vi "CRYSelect result by name.vi"(10 "Result name desired":string, 11 "Result array":T2 {"Margin" format="%.2f"}) -> (0 "Exists?":bool, 3 "Desired Result":T1={"Name"="Test for Signal [L]", "Margin"=nan, "unit"="", "Verdict"=FALSE, "Limit"="", "Max/Min"="", "protected"=FALSE, "Step No."=0, "Test Info"="", "AutoProtect"=FALSE} {"Margin" format="%.2f"})   [LabVIEW 2013]
uses:
  Typedef Control/CRYResult Cluster Array.ctl
  Typedef Control/CRYResult Cluster.ctl
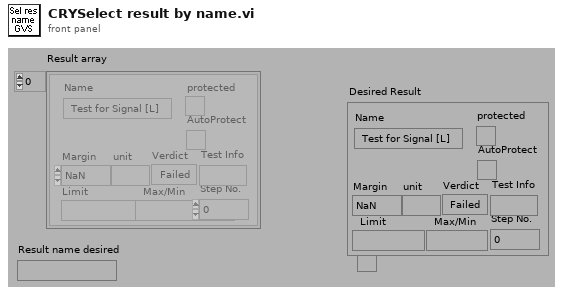
[diagram p1: front panel]
types:
  T1 = typedef "CRYResult Cluster.ctl" = cluster{"Name":string, "Margin":dbl, "unit":string, "Verdict":bool, "Limit":string, "Max/Min":string, "protected":bool, "Step No.":i32, "Test Info":string, "AutoProtect":bool}
  T2 = typedef "CRYResult Cluster Array.ctl" = T1[]
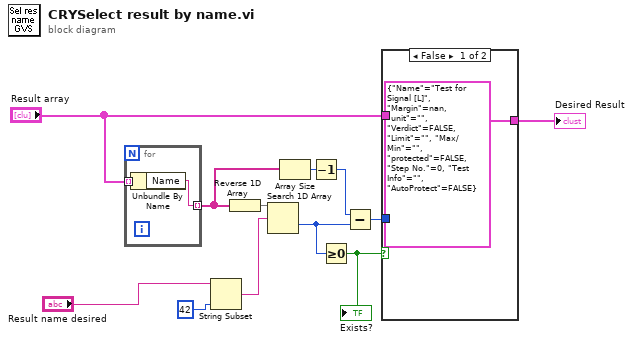
[diagram p0: block diagram]
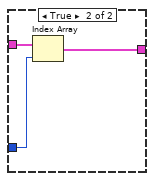
[diagram p2: hidden frame]
diagram:
  n1 = for {
    tunnel: "Result array" -> [w14] mode=indexing
    tunnel: [w13] -> w8 mode=indexing
    n2 = Unbundle By Name(w14) -> ("Name"=w13:string)
  }
  n3 = String Subset(string="Result name desired", length (rest)=42 ("length")) -> (substring=w3:string)  [unwired: 1 in]
  n4 = Reverse 1D Array(array=w8) -> (reversed array=w11:string[])
  n5 = Search 1D Array(1D array=w11, element=w3) -> (index of element=w10:i32)  [unwired: 1 in]
  n6 = Array Size(array=w8) -> (size(s)=w7:i32)
  n7 = Decrement(x=w7) -> (x-1=w6:i32)
  n8 = Greater Or Equal To 0?(x=w10) -> (x >= 0?=w12:bool)
  "Exists?" <- w12
  n9 = Subtract(x=w6, y=w10) -> (x-y=w9:i32)
  n10 = case shown="False" w12 {
    tunnel: "Result array" -> [_ w18]
    tunnel: w9 -> [_ w17]
    tunnel: [T1 {"Name"="Test for Signal [L]", "Margin"=nan, "unit"="", "Verdict"=FALSE, "Limit"="", "Max/Min"="", "protected"=FALSE, "Step No."=0, "Test Info"="", "AutoProtect"=FALSE} ("Result") w16] -> w1
    frame False {
    }
    frame True {
      n11 = Index Array(array=w18, index=w17) -> (element=w16:T1)
    }
  }
  "Desired Result" <- w1
